vi "getDataSubset.vi"(8 "error in (no error)":errorcluster, 10 "Length":i32, 11 "FrameParser in":refnum<class "DynamicFrameParser.lvclass">) -> (0 "error out":errorcluster, 2 "Data":u8[](array[numeric]), 3 "FrameParser out":refnum<class "DynamicFrameParser.lvclass">)   [LabVIEW 2015, in "RTModbus.lvlib" / "DynamicFrameParser.lvclass"]
uses:
  DynamicFrameParser.lvclass
  DynamicFrameParser.lvclass/DynamicFrameParser.ctl
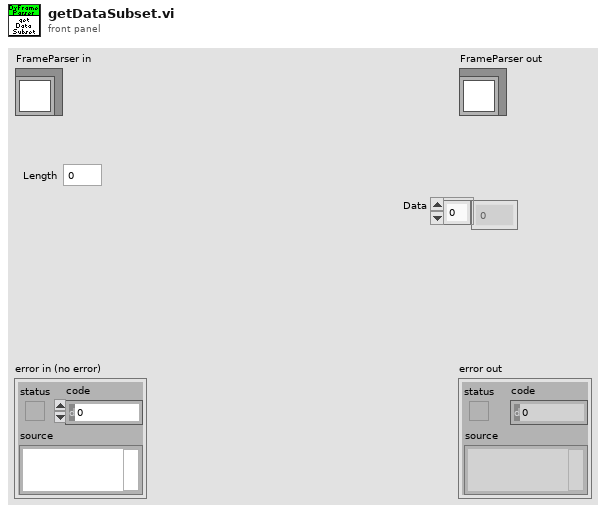
[diagram p1: front panel]
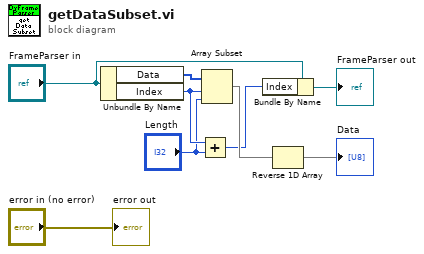
[diagram p0: block diagram]
diagram:
  n1 = Unbundle By Name("FrameParser in") -> ("Data"=w9:u8[], "Index"=w4:i32)
  n2 = Add(x=w4, y="Length") -> (x+y=w2:i32)
  n3 = Array Subset(array=w9, index=w4, length="Length") -> (w7:u8[])
  n4 = Bundle By Name(cluster="FrameParser in", "Index"=w2) -> (→"FrameParser out":refnum<class "DynamicFrameParser.lvclass">)
  n5 = Reverse 1D Array(array=w7) -> (reversed array=→"Data":u8[])
  "error out" <- "error in (no error)"
